vi "niFpgaScaledWinInsideSCTL.vi"(0 "real data in":fxp<+/-,24,1>, 1 "reset":bool, 5 "imaginary data in":fxp<+/-,24,1>, 9 "input valid":bool, 12 "ready for output":bool) -> (3 "data index":u16, 4 "real data out":fxp<+/-,24,-1>, 6 "imaginary data out":fxp<+/-,24,-1>, 10 "output valid":bool, 14 "ready for input":bool)   [LabVIEW 2017]
uses:
  <vilib>/rvi/FXPMathLib/basic elements/FxpDiscreteDelay/XNode/nifxpmath_DiscreteDelay.xnode
  <vilib>/rvi/FXPMathLib/FxpMul/XNode/nifxpmath_Multiplier.xnode
  <vilib>/rvi/FXPMathLib/sim/FxpSim.dll
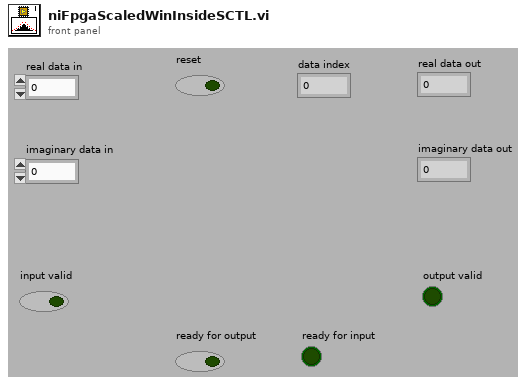
[diagram p1: front panel]
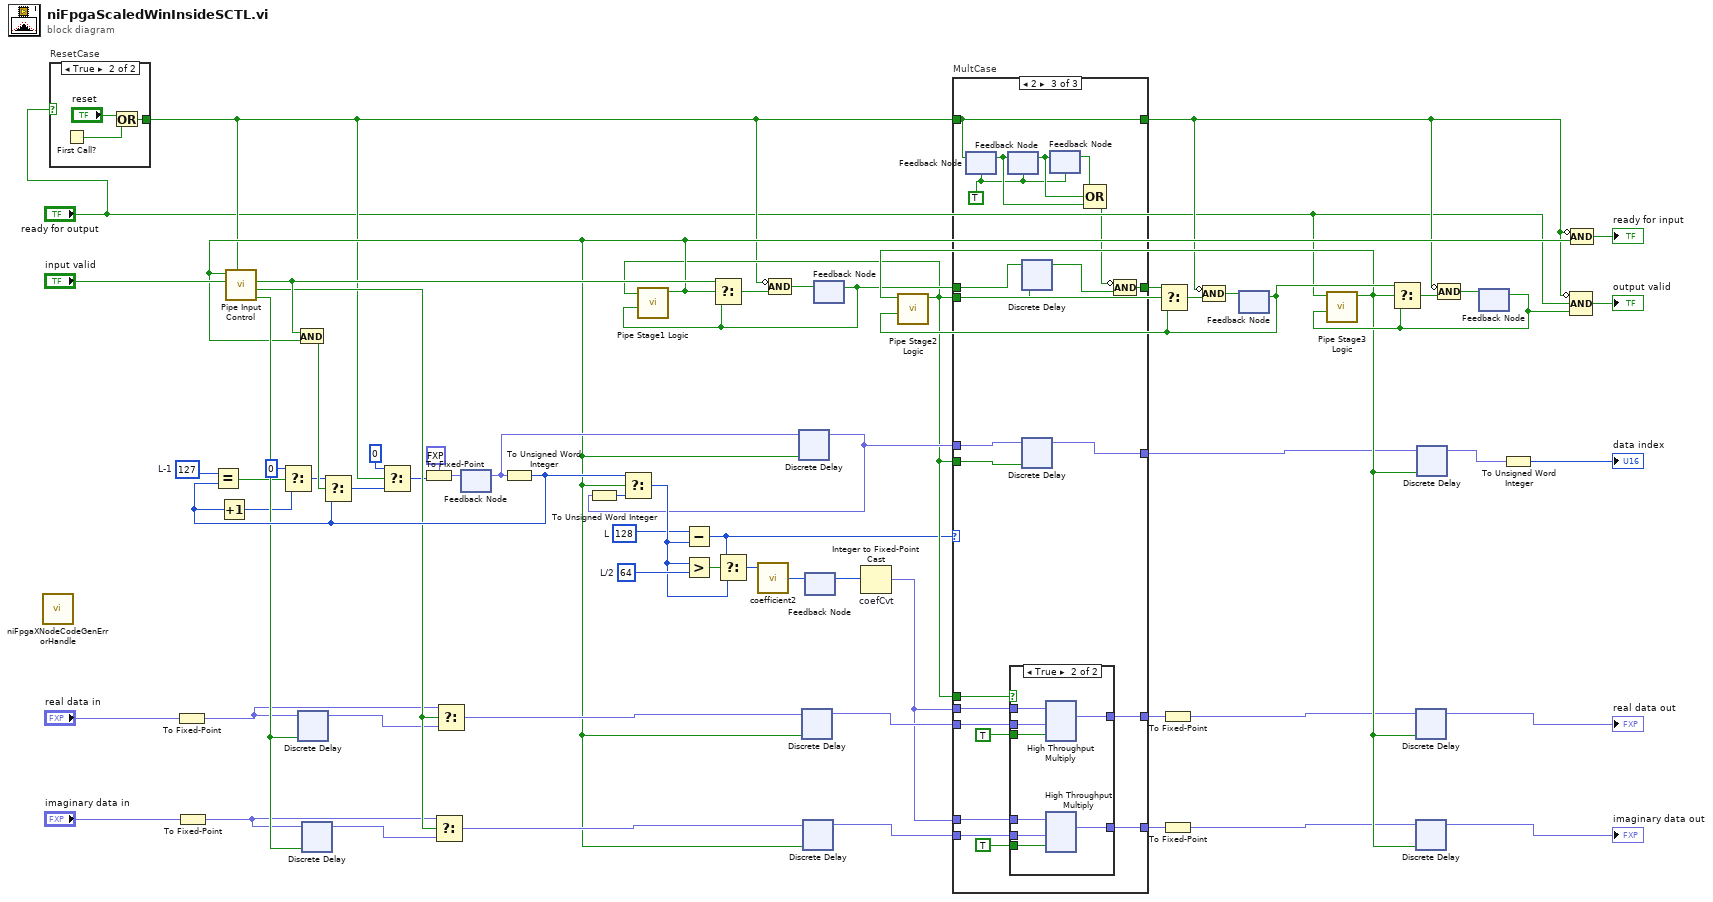
[diagram p0: block diagram]
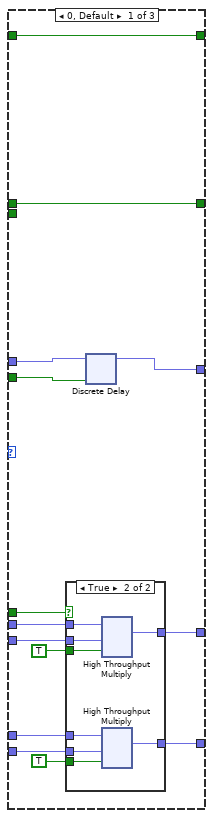
[diagram p2: hidden frame]
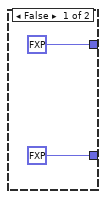
[diagram p3: hidden frame]
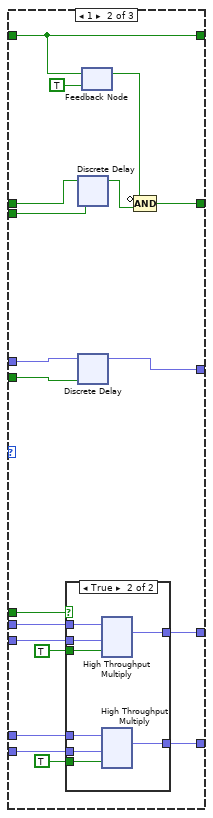
[diagram p4: hidden frame]
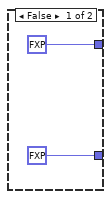
[diagram p5: hidden frame]
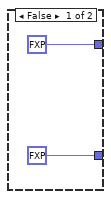
[diagram p6: hidden frame]
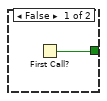
[diagram p7: hidden frame]
diagram:
  w10 = u16 127  # L-1
  w48 = u16 128  # L
  w53 = u16 64  # L/2
  n1 = call <vilib>:"niFpgaXNodeCodeGenErrorHandle.vi"() -> ()  [unwired: 1 in]
  n2 = case "ResetCase" shown="True" "ready for output" {
    tunnel: [w66 w67] -> w24
    frame False {
      n3 = First Call?() -> (First Call?: T/F=w66:bool)
    }
    frame True {
      n4 = First Call?() -> (First Call?: T/F=w68:bool)
      n5 = Or(x="reset", y=w68) -> (x .or. y?=w67:bool)
    }
  }
  n6 = To Fixed-Point(number="real data in") -> (fixed-point=w6:fxp<+/-,24,1>)  [unwired: 1 in]
  n7 = To Fixed-Point(number="imaginary data in") -> (fixed-point=w4:fxp<+/-,24,1>)  [unwired: 1 in]
  n8 = feedback #1() -> (w33:fxp<+,7,7>)  [unwired: 1 out]
  n9 = To Unsigned Word Integer(number=w33) -> (unsigned 16bit integer=w47:u16)
  n10 = Equal?(x=w10, y=w47) -> (x = y?=w9:bool)
  n11 = Increment(x=w47) -> (x+1=w15:u16)
  n12 = Select(t=u16 0, s=w9, f=w15) -> (s? t:f=w16:u16)
  n13 = feedback #2() -> (w2:i32)  [unwired: 1 out]
  n14 = feedback #3() -> (w27:bool)  [unwired: 1 out]
  n15 = Integer to Fixed-Point Cast "coefCvt"(integer=w2) -> (fixed-point=w1:fxp<+/-,32,32>)  [unwired: 1 in]
  n16 = feedback #4() -> (w58:bool)  [unwired: 1 out]
  n17 = feedback #5() -> (w57:bool)  [unwired: 1 out]
  n18 = call "Pipe Stage3 Logic"("last output valid"=w57, "ready for output"="ready for output") -> ("ready For input"=w34:bool)  [unwired: 9 out]
  n19 = call "Pipe Stage2 Logic"("last output valid"=w58, "ready for output"=w34) -> ("ready For input"=w25:bool)  [unwired: 9 out]
  n20 = call "Pipe Stage1 Logic"("last output valid"=w27, "ready for output"=w25) -> ("ready For input"=w32:bool)  [unwired: 9 out]
  n21 = call "Pipe Input Control"("reset"=w24, "input valid"="input valid", "ready for input"=w32) -> ("input buffer enable"=w41:bool, "Input Mux Sel"=w44:bool, "output valid"=w65:bool)  [unwired: 6 out]
  n22 = And(x=w65, y=w32) -> (x .and. y?=w55:bool)
  n23 = xnode "Discrete Delay"("D"=w6, "enable"=w41) -> ("Q"=w42:fxp<+/-,24,1>)
  n24 = xnode "Discrete Delay"("D"=w4, "enable"=w41) -> ("Q"=w40:fxp<+/-,24,1>)
  n25 = Select(t=w16, s=w55, f=w47) -> (s? t:f=w12:u16)
  n26 = Select(t=u16 0, s=w24, f=w12) -> (s? t:f=w11:u16)
  n27 = To Fixed-Point(fixed-point type=fxp<+,7,7> 0.0 ("LBitMask"), number=w11) -> (fixed-point=w14:fxp<+,7,7>)
  n28 = Select(t=w4, s=w44, f=w40) -> (s? t:f=w38:fxp<+/-,24,1>)
  n29 = Select(t=w6, s=w44, f=w42) -> (s? t:f=w39:fxp<+/-,24,1>)
  n30 = feedback-in #1(w14) -> ()
  n31 = Select(t=w65, s=w32, f=w27) -> (s? t:f=w64:bool)
  n32 = Compound Arithmetic op=AND(invert w24, w64) -> (w63:bool)
  n33 = xnode "Discrete Delay"("D"=w33, "enable"=w32) -> ("Q"=w31:fxp<+,7,7>)
  n34 = To Unsigned Word Integer(number=w31) -> (unsigned 16bit integer=w49:u16)
  n35 = Select(t=w47, s=w32, f=w49) -> (s? t:f=w51:u16)
  n36 = Subtract(x=w48, y=w51) -> (x-y=w7:u16)
  n37 = Greater?(x=w51, y=w53) -> (0:w54:bool)
  n38 = Select(t=w7, s=w54, f=w51) -> (s? t:f=w50:u16)
  n39 = call "coefficient2"("address"=w50) -> ("data out"=w52:i32)  [unwired: 8 in]
  n40 = xnode "Discrete Delay"("D"=w39, "enable"=w32) -> ("Q"=w29:fxp<+/-,24,1>)
  n41 = xnode "Discrete Delay"("D"=w38, "enable"=w32) -> ("Q"=w28:fxp<+/-,24,1>)
  n42 = feedback-in #2(w52) -> ()
  n43 = feedback-in #3(w63) -> ()
  n44 = case "MultCase" shown="2" w7 {
    tunnel: w31 -> [w83 w112 w144]
    tunnel: w25 -> [w82 w111 w143]
    tunnel: [w81 w110 w142] -> w30
    tunnel: w1 -> [w80 w109 w141]
    tunnel: w29 -> [w79 w108 w140]
    tunnel: w1 -> [w78 w107 w139]
    tunnel: w28 -> [w77 w106 w138]
    tunnel: [w71 w95 w125] -> w22
    tunnel: [w72 w96 w126] -> w20
    tunnel: w25 -> [w76 w105 w137]
    tunnel: w27 -> [w75 w103 w136]
    tunnel: [w75 w100 w134] -> w26
    tunnel: w25 -> [_ w99 w133]
    tunnel: w24 -> [w70 w94 w124]
    tunnel: [w70 w94 w124] -> w23
    frame 0, Default {
      n45 = case shown="True" w76 {
        tunnel: w80 -> [_ w93]
        tunnel: w79 -> [_ w92]
        tunnel: [fxp<+,1,1> 0.0 w91] -> w72
        tunnel: w78 -> [_ w90]
        tunnel: w77 -> [_ w89]
        tunnel: [fxp<+,1,1> 0.0 w88] -> w71
        tunnel: TRUE -> [_ w87]
        tunnel: TRUE -> [_ w86]
        frame False {
        }
        frame True {
          n46 = xnode "High Throughput Multiply"("x"=w93, "y"=w92, "input valid"=w87) -> ("x*y"=w91:fxp<+/-,56,33>)  [unwired: 1 in, 2 out]
          n47 = xnode "High Throughput Multiply"("x"=w90, "y"=w89, "input valid"=w86) -> ("x*y"=w88:fxp<+/-,56,33>)  [unwired: 1 in, 2 out]
        }
      }
      n48 = xnode "Discrete Delay"("D"=w83, "enable"=w82) -> ("Q"=w81:fxp<+,7,7>)
    }
    frame 1 {
      n49 = case shown="True" w105 {
        tunnel: w109 -> [_ w122]
        tunnel: w108 -> [_ w121]
        tunnel: [fxp<+,1,1> 0.0 w120] -> w96
        tunnel: w107 -> [_ w119]
        tunnel: w106 -> [_ w118]
        tunnel: [fxp<+,1,1> 0.0 w117] -> w95
        tunnel: TRUE -> [_ w116]
        tunnel: TRUE -> [_ w115]
        frame False {
        }
        frame True {
          n50 = xnode "High Throughput Multiply"("x"=w122, "y"=w121, "input valid"=w116) -> ("x*y"=w120:fxp<+/-,56,33>)  [unwired: 1 in, 2 out]
          n51 = xnode "High Throughput Multiply"("x"=w119, "y"=w118, "input valid"=w115) -> ("x*y"=w117:fxp<+/-,56,33>)  [unwired: 1 in, 2 out]
        }
      }
      n52 = xnode "Discrete Delay"("D"=w103, "enable"=w99) -> ("Q"=w102:bool)
      n53 = xnode "Discrete Delay"("D"=w112, "enable"=w111) -> ("Q"=w110:fxp<+,7,7>)
      n54 = feedback-in #6(w94) -> ()
      n55 = feedback #6(TRUE ("First Call?: T/F")) -> (w101:bool)
      n56 = Compound Arithmetic op=AND(invert w101, w102) -> (w100:bool)
    }
    frame 2 {
      w123 = TRUE ("First Call?: T/F")
      n57 = feedback-in #7(w124) -> ()
      n58 = feedback #7(w123) -> (w130:bool)
      n59 = feedback-in #8(w130) -> ()
      n60 = feedback #8(w123) -> (w131:bool)
      n61 = case shown="True" w137 {
        tunnel: w141 -> [_ w154]
        tunnel: w140 -> [_ w153]
        tunnel: [fxp<+,1,1> 0.0 w152] -> w126
        tunnel: w139 -> [_ w151]
        tunnel: w138 -> [_ w150]
        tunnel: [fxp<+,1,1> 0.0 w149] -> w125
        tunnel: TRUE -> [_ w148]
        tunnel: TRUE -> [_ w147]
        frame False {
        }
        frame True {
          n62 = xnode "High Throughput Multiply"("x"=w154, "y"=w153, "input valid"=w148) -> ("x*y"=w152:fxp<+/-,56,33>)  [unwired: 1 in, 2 out]
          n63 = xnode "High Throughput Multiply"("x"=w151, "y"=w150, "input valid"=w147) -> ("x*y"=w149:fxp<+/-,56,33>)  [unwired: 1 in, 2 out]
        }
      }
      n64 = xnode "Discrete Delay"("D"=w136, "enable"=w133) -> ("Q"=w135:bool)
      n65 = xnode "Discrete Delay"("D"=w144, "enable"=w143) -> ("Q"=w142:fxp<+,7,7>)
      n66 = feedback-in #9(w131) -> ()
      n67 = feedback #9(w123) -> (w132:bool)
      n68 = Compound Arithmetic op=OR(w132, w131, w130) -> (w129:bool)
      n69 = Compound Arithmetic op=AND(invert w129, w135) -> (w134:bool)
    }
  }
  n70 = Select(t=w26, s=w25, f=w58) -> (s? t:f=w62:bool)
  n71 = To Fixed-Point ("MultCast")(number=w20) -> (fixed-point=w19:fxp<+/-,24,-1>)  [unwired: 1 out]
  n72 = To Fixed-Point ("MultCast")(number=w22) -> (fixed-point=w21:fxp<+/-,24,-1>)  [unwired: 1 out]
  n73 = Compound Arithmetic op=AND(invert w23, w62) -> (w61:bool)
  n74 = feedback-in #4(w61) -> ()
  n75 = Select(t=w58, s=w34, f=w57) -> (s? t:f=w59:bool)
  n76 = xnode "Discrete Delay"("D"=w19, "enable"=w34) -> ("Q"=→"real data out":fxp<+/-,24,-1>)
  n77 = xnode "Discrete Delay"("D"=w21, "enable"=w34) -> ("Q"=→"imaginary data out":fxp<+/-,24,-1>)
  n78 = xnode "Discrete Delay"("D"=w30, "enable"=w34) -> ("Q"=w35:fxp<+,7,7>)
  n79 = Compound Arithmetic op=AND(invert w23, w59) -> (w60:bool)
  n80 = feedback-in #5(w60) -> ()
  n81 = To Unsigned Word Integer(number=w35) -> (unsigned 16bit integer=→"data index":u16)
  n82 = Compound Arithmetic op=AND(invert w23, "ready for output", w57) -> (→"output valid":bool)
  n83 = Compound Arithmetic op=AND(invert w23, w32) -> (→"ready for input":bool)
